vi "Math-Sigmoid.vi"(2 "Parameter":dbl, 3 "X0":dbl, 4 "X":dbl) -> (0 "Y":dbl)   [LabVIEW 2015]
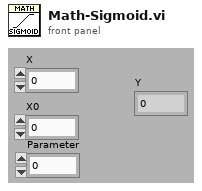
[diagram p1: front panel]
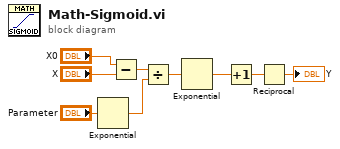
[diagram p0: block diagram]
diagram:
  n1 = Exponential(1:"Parameter") -> (0:w5:dbl)
  n2 = Subtract(x="X0", y="X") -> (x-y=w2:dbl)
  n3 = Divide(x=w2, y=w5) -> (x/y=w6:dbl)
  n4 = Exponential(1:w6) -> (0:w7:dbl)
  n5 = Increment(x=w7) -> (x+1=w8:dbl)
  n6 = Reciprocal(x=w8) -> (1/x=→"Y":dbl)
